vi "Simple Latch.vi"(7 "Reset":bool, 11 "Input":bool) -> (3 "Output":bool)   [LabVIEW 2022 SP3, in "hse-misc.lvlib"]
doc: "A simple boolean latch with reset functionality.\n\n____\nHAMPEL SOFTWARE ENGINEERING v3.8.0 (2023-12-18 14:41)"
uses:
  hse-misc.lvlib
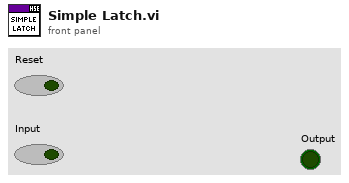
[diagram p1: front panel]
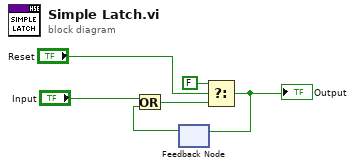
[diagram p0: block diagram]
diagram:
  n1 = feedback #1() -> (w5:bool)  [unwired: 1 in]
  n2 = Or(x="Input", y=w5) -> (x .or. y?=w3:bool)
  n3 = Select(t=FALSE, s="Reset", f=w3) -> (s? t:f=w2:bool)
  "Output" <- w2
  n4 = feedback-in #1(w2) -> ()
